vi "rectangle_to_ROI.vi"(1 "ROI Type flag":bool, 2 "ROI bounds":i32[](array[numeric])) -> (0 "ROI":T1)   [LabVIEW 2015]
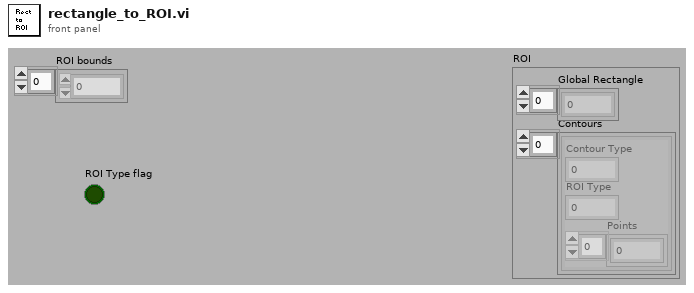
[diagram p1: front panel]
types:
  T1 = cluster{"Global Rectangle":i32[], "Contours":cluster{"Contour Type":u32, "ROI Type":u32, "Points":i32[]}[]}
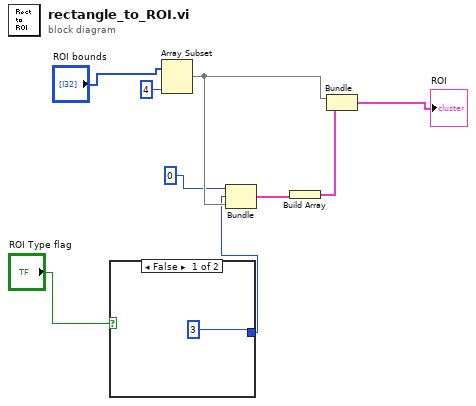
[diagram p0: block diagram]
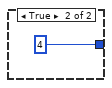
[diagram p2: hidden frame]
diagram:
  n1 = case shown="False" "ROI Type flag" {
    tunnel: [3 4] -> w2
    frame False {
    }
    frame True {
    }
  }
  n2 = Array Subset(array="ROI bounds", length=4) -> (w5:i32[])  [unwired: 1 in]
  n3 = Bundle(0, w2, w5) -> (w7:cluster{i32, i32, i32[]})  [unwired: 1 in]
  n4 = Build Array(w7) -> (w6:cluster{i32, i32, i32[]}[])
  n5 = Bundle(w5, w6) -> (→"ROI":cluster{i32[], cluster{i32, i32, i32[]}[]})  [unwired: 1 in]
